vi "Send to DAQ.vi"(6 "File?":bool, 7 "Port Number":u16, 8 "error in (no error)":errorcluster, 9 "Data":variant, 10 "Data Name":string, 11 "Father of all uServices in":refnum<class "Father of all uServices.lvclass">) -> (0 "error out":errorcluster, 3 "Father of all uServices out":refnum<class "Father of all uServices.lvclass">)   [LabVIEW 2026, in "TALOS.lvlib" / "Father of all uServices.lvlib" / "Father of all uServices.lvclass"]
doc: "Use this VI to send data to the DAQ. If an entire file is needed to be sent, set File?=True and provide the path of the file to be sent in the Data field."
uses:
  Father of all uServices.lvclass
  C:/LabVIEW Code/TALOS/talos/Ancestor/Ancestor/Ancestor.lvclass
  C:/LabVIEW Code/TALOS/builds/Actor Framework PPL/Actor Framework.lvlibp/1abvi3w/vi.lib/ActorFramework/Actor/Actor.lvclass
  Ancestor/Ancestor/Ancestor.lvclass/Ancestor.ctl
  Interfaces/DAQ Communication/DAQ Sender Payload.ctl
  Interfaces/DAQ Communication/DAQ Message.ctl
  Guardian/Guardian Messages/Message to uService Msg/Message to uService Msg.lvclass/Message to uService Msg.ctl
  Ancestor/Ancestor/Read ID.vi
  Guardian/Guardian Messages/Message to uService Msg/Send Message to uService.vi
  Support VIs/Substitute Error.vi
  Support VIs/Generate Error.vi
  FGV/Error Memory/Get Error Description.vi
  Support VIs/Get PC name.vi
  Support VIs/Get Class Name.vi
  <vilib>/Utility/error.llb/Clear Errors.vi
  FGV/Error Memory/Error Memory Core.vi
  <vilib>/AdvancedString/Delimited String to 1D String Array.vi
  <vilib>/AdvancedString/Delimited String to 1D String Array (string).vi
  Support VIs/Circus Root Path.vi
  FGV/Error Memory/Error Crt Lvl checker.vi
  FGV/Error Memory/Error Memory Core.vi/40c8088d-b597-4017-91af-faa98e00292e.vi
  FGV/Error Memory/Error Memory Core.vi/d4a3ab98-063c-4e44-b43d-fbdcfe6c2be2.vi
  Support VIs/Global Memory.vi
  builds/Actor Framework PPL/Actor Framework.lvlibp/1abvi3w/vi.lib/ActorFramework/Actor/Read Caller Enqueuer.vi
  builds/Actor Framework PPL/Actor Framework.lvlibp/1abvi3w/vi.lib/ActorFramework/Message Enqueuer/Enqueue.vi
  <vilib>/Utility/LVClass/Get LV Class Name.vi
  Support VIs/Is in Packed Library.vi
  Support VIs/TALOS Root path.vi
  Support VIs/Read CSV worksheet.vi
  Support VIs/Global Constants.vi
  <vilib>/Utility/error.llb/General Error Handler.vi
  Support VIs/Error Log.vi
  Guardian/Guardian Messages/Message to uService Msg/Message to uService Msg.lvclass
  Ancestor/Ancestor/Ancestor.lvclass
  <vilib>/Comparison/Equal/Equal Functor/Equal Functor.lvclass
  TALOS.lvlib
  Interfaces/DAQ Communication/DAQ Communication.lvclass
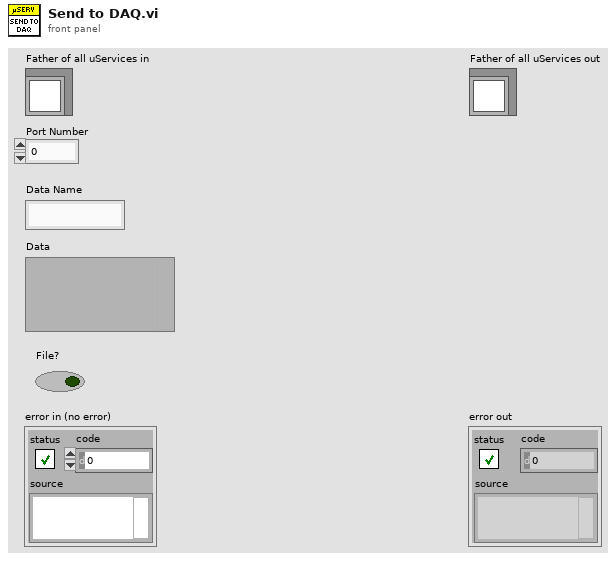
[diagram p1: front panel]
types:
  T1 = typedef "TALOS.lvlib/Interfaces.lvlib/DAQ Communication.lvclass/DAQ Sender Payload.ctl" = cluster{"Sender uS":string, "DAQ Message":T2, "DAQ Address":cluster{"Port":u16, "Path":string}}
  T2 = typedef "TALOS.lvlib/Interfaces.lvlib/DAQ Communication.lvclass/DAQ Message.ctl" = cluster{"Path":string, "Port":u16, "Data Name":string, "Data":variant, "File?":bool, "Timestamp":timestamp}
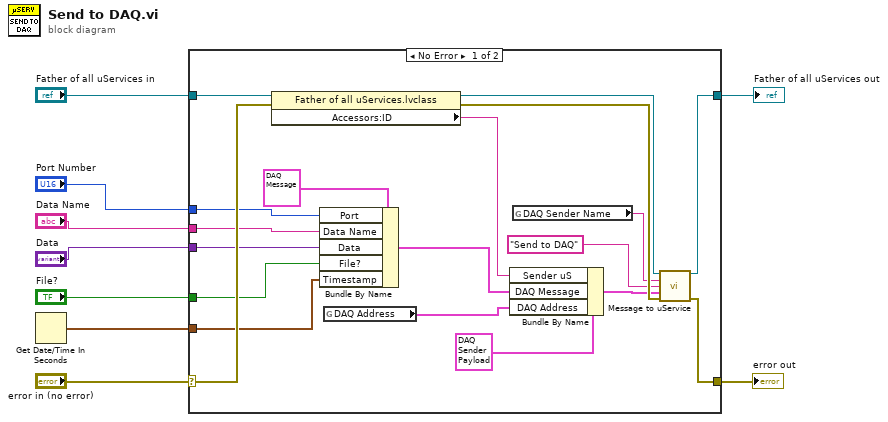
[diagram p0: block diagram]
diagram:
  n1 = Get Date/Time In Seconds() -> (seconds since 1Jan1904=w1:timestamp)
  n2 = case shown="No Error" "error in (no error)" {
    selector: "error in (no error)" -> [w28 w29]
    tunnel: [w26 w29] -> w8
    tunnel: "Father of all uServices in" -> [w25 w30]
    tunnel: [w24 w30] -> w6
    tunnel: "Port Number" -> [w21 _]
    tunnel: "Data Name" -> [w20 _]
    tunnel: "Data" -> [w19 _]
    tunnel: "File?" -> [w18 _]
    tunnel: w1 -> [w16 _]
    frame No Error {
      n3 = property class="Father of all uServices.lvclass"(reference=w25, error in=w28) -> (reference out=w14:refnum<class "Father of all uServices.lvclass">, error out=w27:errorcluster, "Accessors:ID"=w12:string)
      n4 = Bundle By Name(cluster=T2 {"Path"="", "Port"=0, "Data Name"="", "Data"=variant, "File?"=FALSE, "Timestamp"=timestamp(0 s since 1904-01-01)} ("DAQ Message"), "Port"=w21, "Data Name"=w20, "Data"=w19, "File?"=w18, "Timestamp"=w16) -> (w11:T2)
      n5 = global read "Global Memory.vi" "DAQ Address"() -> (w10:cluster{"Port":u16, "Path":string})
      n6 = Bundle By Name(cluster=T1 {"Sender uS"="", "DAQ Message"={"Path"="", "Port"=0, "Data Name"="", "Data"=variant, "File?"=FALSE, "Timestamp"=timestamp(0 s since 1904-01-01)}, "DAQ Address"={"Port"=0, "Path"=""}} ("DAQ Sender Payload"), "Sender uS"=w12, "DAQ Message"=w11, "DAQ Address"=w10) -> (w15:T1)
      n7 = global read "Global Memory.vi" "DAQ Sender Name"() -> (w17:string)
      n8 = call "Message to uService.vi"("Father of all uServices in"=w14, "uService ID"=w17, "Message"="Send to DAQ", "Data"=w15, "error in (no error)"=w27) -> ("Father of all uServices out"=w24:refnum<class "Father of all uServices.lvclass">, "error out"=w26:errorcluster)  [unwired: 9 in]
    }
    frame Error {
    }
  }
  "error out" <- w8
  "Father of all uServices out" <- w6
